vi "FeedbackNotesMarcoGonzalez.vi"() -> ()   [LabVIEW 2012]
panel:
  in  "Factorial 2":dbl
  out "Result 2":dbl
  in  "Factorial":dbl
  out "Result":dbl
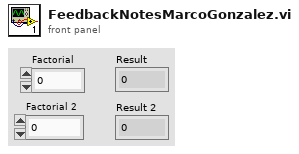
[diagram p1: front panel]
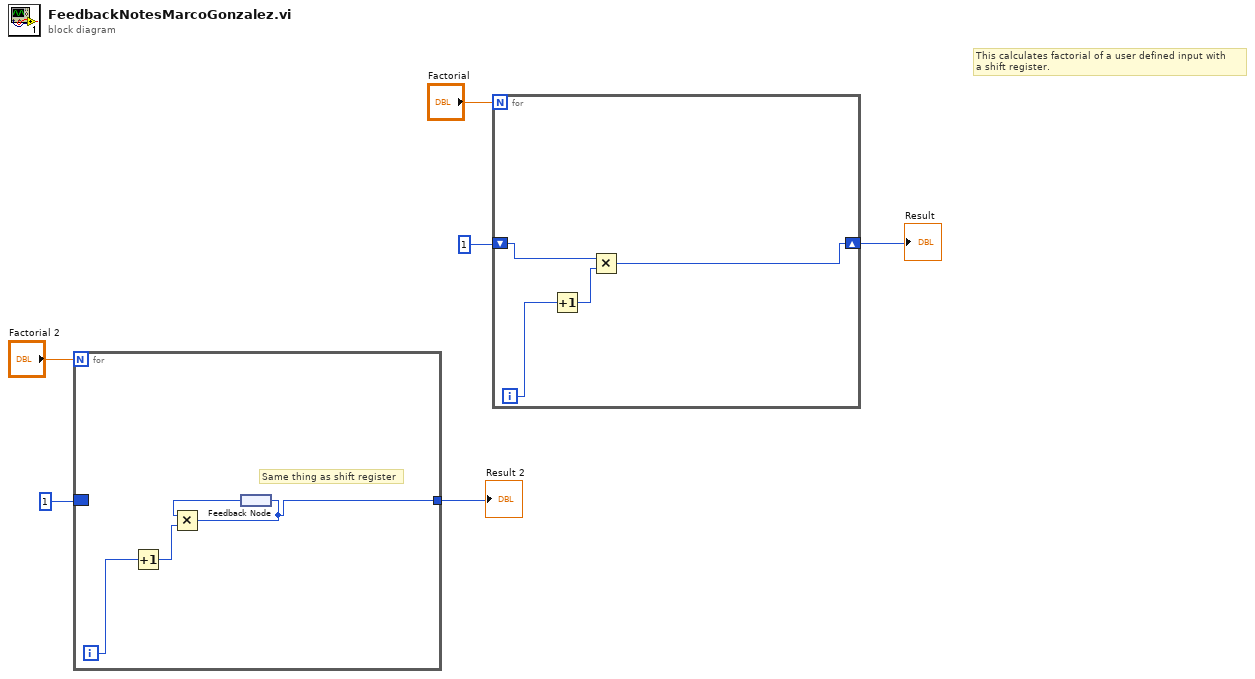
[diagram p0: block diagram]
diagram:
  # "This calculates factorial of a user defined input with \na shift register."
  n1 = for {
    N: "Factorial 2" -> [_]
    border: 1 -> [_]
    tunnel: [w7] -> w1
    i -> [w9]
    # "Same thing as shift register"
    n2 = Increment(x=w9) -> (x+1=w10:i32)
    n3 = feedback #1() -> (w8:i32)
    n4 = Multiply(x=w8, y=w10) -> (x*y=w7:i32)
    n5 = feedback-in #1(w7) -> ()
  }
  "Result 2" <- w1
  n6 = for {
    N: "Factorial" -> [_]
    shift-right: [w11] -> w5
    shift-left: 1 -> [w13]
    i -> [w12]
    n7 = Increment(x=w12) -> (x+1=w14:i32)
    n8 = Multiply(x=w13, y=w14) -> (x*y=w11:i32)
  }
  "Result" <- w5
